vi "Display Setup.vi"(0 "VISA resource name":refnum<visa-resource-name>, 5 "Enable Display (T: Enable)":bool=TRUE, 7 "Display Mode (0: Normal)":u16(ring) items=["Normal", "Text"], 9 "Text Input":string, 11 "error in (no error)":errorcluster) -> (4 "VISA resource name out":refnum<visa-resource-name>, 15 "error out":errorcluster)   [LabVIEW 2019, in "Agilent 681x Series.lvlib"]
doc: "Configures the display settings of the instrument."
uses:
  <instrlib>/Agilent 681x Series/Agilent 681x Series.lvlib
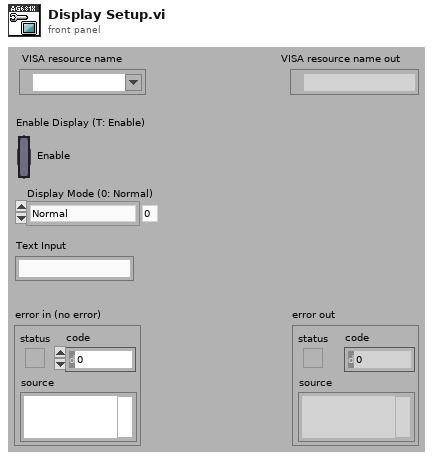
[diagram p1: front panel]
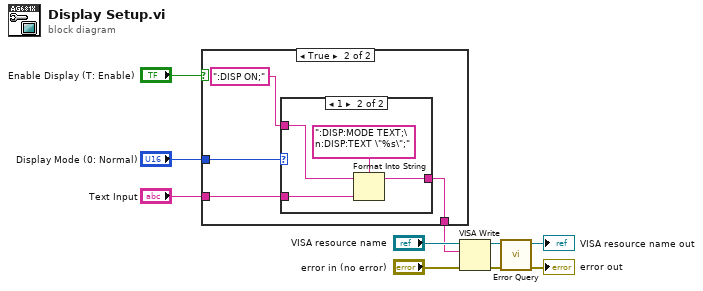
[diagram p0: block diagram]
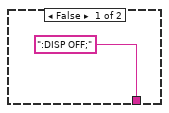
[diagram p2: hidden frame]
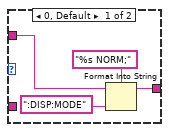
[diagram p3: hidden frame]
diagram:
  n1 = case shown="True" "Enable Display (T: Enable)" {
    tunnel: "Display Mode (0: Normal)" -> [_ w15]
    tunnel: [":DISP OFF;" ("output string") w12] -> w6
    tunnel: "Text Input" -> [_ w13]
    frame False {
    }
    frame True {
      n2 = case shown="1" w15 {
        tunnel: ":DISP ON;" -> [w19 w21]
        tunnel: w13 -> [_ w23]
        tunnel: [w16 w20] -> w12
        frame 0, Default {
          n3 = Format Into String(format string="%s NORM;", initial string=w19, ":DISP:MODE" ("format string")) -> (resulting string=w16:string)  [unwired: 1 in, 1 out]
        }
        frame 1 {
          n4 = Format Into String(format string=":DISP:MODE TEXT;\n:DISP:TEXT \"%s\";", initial string=w21, w23) -> (resulting string=w20:string)  [unwired: 1 in, 1 out]
        }
      }
    }
  }
  n5 = VISA Write(VISA resource name="VISA resource name", write buffer=w6, error in (no error)="error in (no error)") -> (VISA resource name out=w3:refnum<visa-resource-name>, error out=w4:errorcluster)  [unwired: 1 out]
  n6 = call <instrlib>:"Error Query.vi"("error in (no error)"=w4, "VISA resource name"=w3) -> ("error out"=→"error out":errorcluster, "VISA resource name out"=→"VISA resource name out":refnum<visa-resource-name>)  [unwired: 6 in, 2 out]
